vi "ini_object_load_vector.vi"(7 "generate error if unsuppoted data type (true)":bool=TRUE, 8 "error in":errorcluster, 10 "objects to save":T1[](array[typedef]), 11 "refnum in":T2) -> (0 "error out":errorcluster, 3 "refnum out":T2)   [LabVIEW 2018]
uses:
  <vilib>/Utility/config.llb/Config Data RefNum.ctl
  ini_parse_row.ctl
  <vilib>/Utility/config.llb/NI_LVConfig.lvlib
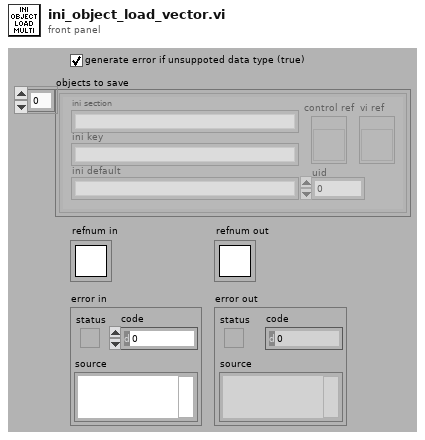
[diagram p1: front panel]
types:
  T1 = typedef "ini_parse_row.ctl" = cluster{"ini section":string, "ini key":string, "ini default":string, "control ref":refnum<vi>, "uid":i32, "vi ref":refnum<vi>}
  T2 = typedef "NI_LVConfig.lvlib/Config Data RefNum.ctl" = refnum<k1>
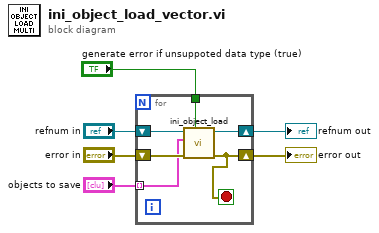
[diagram p0: block diagram]
diagram:
  n1 = for {
    tunnel: "generate error if unsuppoted data type (true)" -> [w9]
    shift-right: [w10] -> w3
    shift-left: "refnum in" -> [w11]
    shift-right: [w7] -> w4
    shift-left: "error in" -> [w12]
    tunnel: "objects to save" -> [w8] mode=indexing
    stop <- w7 stop-if-true
    n2 = call "ini_object_load.vi"("generate error if unsuppoted data type (true)"=w9, "error in"=w12, "auto ini row"=w8, "refnum in"=w11) -> ("error out"=w7:errorcluster, "refnum out"=w10:T2)  [unwired: 6 in]
  }
  "error out" <- w4
  "refnum out" <- w3
